vi "Read String.vi"(8 "error in (no error)":errorcluster, 11 "Serial in":refnum<class "Serial.lvclass">) -> (0 "error out":errorcluster, 1 "Bytes Read":i32, 2 "String Read":string, 3 "Serial out":refnum<class "Serial.lvclass">)   [LabVIEW 2015, in "Serial.lvclass"]
doc: "Serial.lvclass:Read String.vi\n\nThis VI reads the a string of data from a serial port.\n\nInstrument Communication Module Version 1.0\nJuly, 2017 Original Code Consulting David Thomson\n www.originalcode.com"
uses:
  Serial.lvclass
  Serial.lvclass/Serial.ctl
panel:
  out "String Read":string
  out "String Read":string
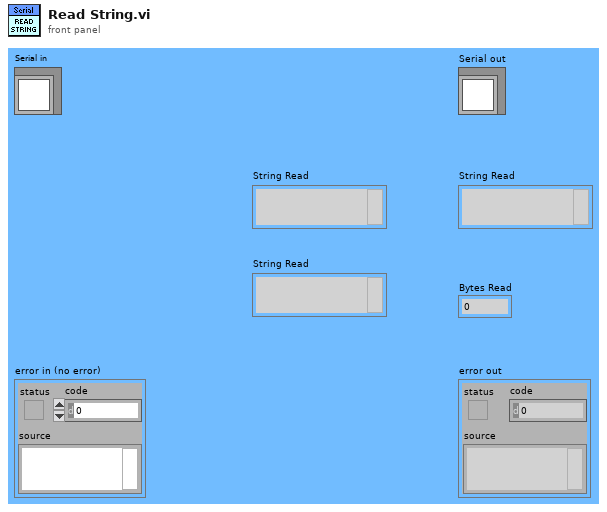
[diagram p1: front panel]
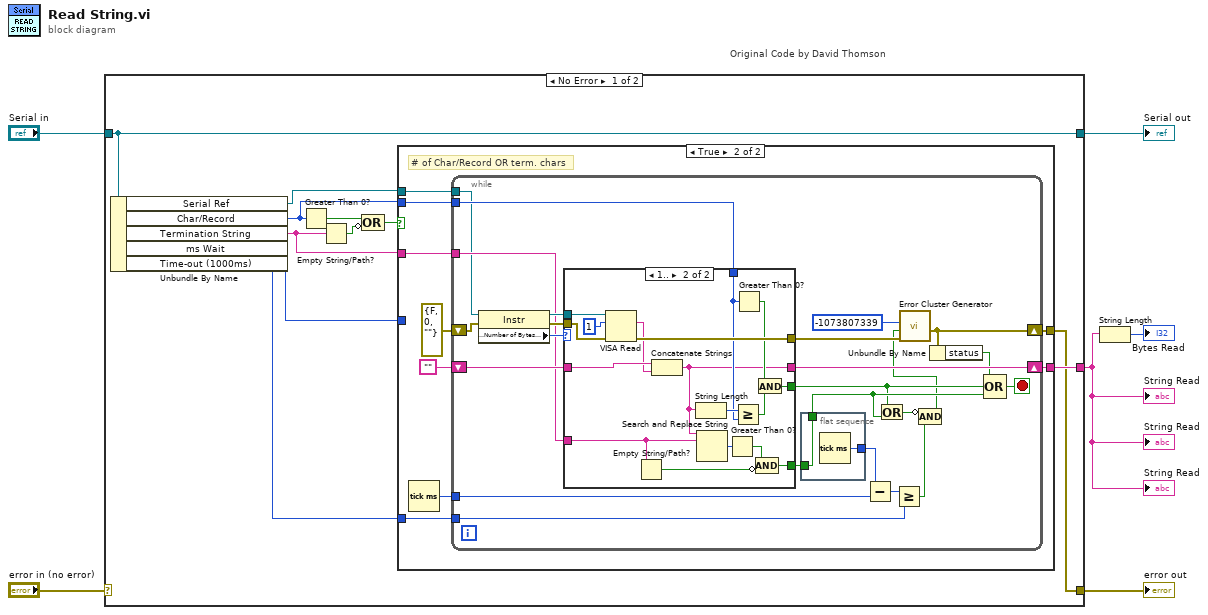
[diagram p0: block diagram]
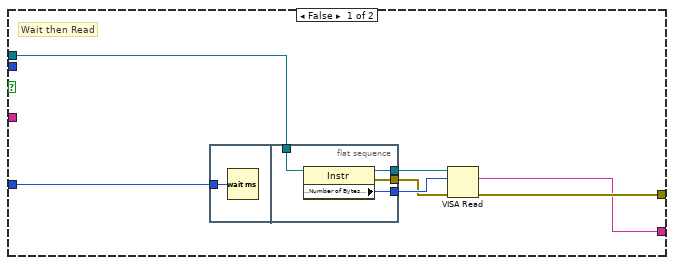
[diagram p2: hidden frame]
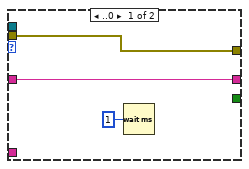
[diagram p3: hidden frame]
diagram:
  n1 = case "Original Code by David Thomson" shown="No Error" "error in (no error)" {
    selector: "error in (no error)" -> [_ w86]
    tunnel: [w7 w86] -> w5
    tunnel: [w17 w85] -> w3
    tunnel: "Serial in" -> [w17 w85]
    tunnel: [w9 _] -> w1
    frame No Error {
      n2 = Unbundle By Name(w17) -> ("Serial Ref"=w12:refnum<visa-resource-name>, "Char/Record"=w13:i32, "Termination String"=w11:string, "ms Wait"=w8:u32, "Time-out (1000ms)"=w10:u32)
      n3 = Greater Than 0?(x=w13) -> (x > 0?=w15:bool)
      n4 = Empty String/Path?(string/path=w11) -> (empty?=w14:bool)
      n5 = Compound Arithmetic op=OR(w15, invert w14) -> (w16:bool)
      n6 = case shown="True" w16 {
        tunnel: w13 -> [_ w38]
        tunnel: w12 -> [w18 w37]
        tunnel: w11 -> [_ w36]
        tunnel: w10 -> [_ w32]
        tunnel: [w19 w31] -> w9
        tunnel: w8 -> [w21 _]
        tunnel: [w20 w30] -> w7
        frame False {
          # "Wait then Read"
          n7 = flat-sequence {
            tunnel: w21 -> [w25]
            tunnel: [w29] -> w24
            tunnel: [w28] -> w23
            tunnel: [w27] -> w22
            tunnel: w18 -> [w26]
            frame #0 {
              n8 = Wait (ms)(milliseconds to wait=w25) -> ()  [unwired: 1 out]
            }
            frame #1 {
              n9 = property class="Instr"(reference=w26) -> (reference out=w29:refnum<visa-resource-name>, error out=w27:errorcluster, "Serial Settings:Number of Bytes at Serial Port"=w28:u32)  [unwired: 1 in]
            }
          }
          n10 = VISA Read(VISA resource name=w24, byte count=w23, error in (no error)=w22) -> (read buffer=w19:string, error out=w20:errorcluster)  [unwired: 2 out]
        }
        frame True {
          # "# of Char/Record OR term. chars"
          n11 = Tick Count (ms)() -> (millisecond timer value=w33:u32)
          n12 = while {
            shift-right: [w47] -> w30
            shift-left: errorcluster {"status"=FALSE, "code"=0, "source"=""} ("error out") -> [w40]
            shift-right: [w58] -> w31
            shift-left: "" -> [w59]
            tunnel: w38 -> [w55]
            tunnel: w36 -> [w54]
            tunnel: w33 -> [w51]
            tunnel: w32 -> [w49]
            tunnel: w37 -> [w39]
            stop <- w57 stop-if-true
            n13 = property class="Instr"(reference=w39, error in=w40) -> (reference out=w61:refnum<visa-resource-name>, error out=w60:errorcluster, "Serial Settings:Number of Bytes at Serial Port"=w62:u32)
            n14 = case shown="1.." w62 {
              tunnel: w61 -> [_ w84]
              tunnel: w60 -> [w66 w82]
              tunnel: [w66 w81] -> w48
              tunnel: w59 -> [w67 w80]
              tunnel: [w67 w72] -> w58
              tunnel: w55 -> [_ w74]
              tunnel: [_ w75] -> w43
              tunnel: w54 -> [_ w68]
              tunnel: [_ w71] -> w53
              frame ..0 {
                n15 = Wait (ms)(milliseconds to wait=u32 1) -> ()  [unwired: 1 out]
              }
              frame 1.. {
                n16 = VISA Read(VISA resource name=w84, byte count=u32 1, error in (no error)=w82) -> (read buffer=w79:string, error out=w81:errorcluster)  [unwired: 2 out]
                n17 = Empty String/Path?(string/path=w68) -> (empty?=w73:bool)
                n18 = Concatenate Strings(w80, w79) -> (w72:string)
                n19 = String Length(string=w72) -> (length=w76:i32)
                n20 = Search and Replace String(input string=w72, search string=w68) -> (number of replacements=w70:i32)  [unwired: 1 in, 8 out]
                n21 = Greater Than 0?(x=w70) -> (x > 0?=w69:bool)
                n22 = Greater Or Equal?(x=w76, y=w74) -> (x >= y?=w77:bool)
                n23 = Greater Than 0?(x=w74) -> (x > 0?=w78:bool)
                n24 = And(x=w78, y=w77) -> (x .and. y?=w75:bool)
                n25 = Compound Arithmetic op=AND(w69, invert w73) -> (w71:bool)
              }
            }
            n26 = flat-sequence {
              tunnel: w53 -> [w63]
              tunnel: [w64] -> w52
              tunnel: [w63] -> w44
              frame #0 {
                n27 = Tick Count (ms)() -> (millisecond timer value=w64:u32)
              }
            }
            n28 = Subtract(x=w52, y=w51) -> (x-y=w50:u32)
            n29 = Or(x=w43, y=w44) -> (x .or. y?=w42:bool)
            n30 = Greater Or Equal?(x=w50, y=w49) -> (x >= y?=w45:bool)
            n31 = Compound Arithmetic op=AND(invert w42, w45) -> (w41:bool)
            n32 = call "Error Cluster Generator.vi"("error in"=w48, "Error (T)"=w41, "code"=-1073807339) -> ("error out"=w47:errorcluster)  [unwired: 1 in, 3 out]
            n33 = Unbundle By Name(w47) -> ("status"=w56:bool)
            n34 = Compound Arithmetic op=OR(w56, w43, w44) -> (w57:bool)
          }
        }
      }
    }
    frame Error {
    }
  }
  "error out" <- w5
  "Serial out" <- w3
  "String Read" <- w1
  "String Read" <- w1
  "String Read" <- w1
  n35 = String Length(string=w1) -> (length=→"Bytes Read":i32)
